vi "Main_FFT.vi"() -> ()   [LabVIEW 2026]
doc: "This template is for the Queued Message Handler design pattern.\n\nThe Event Handling Loop generates messages based on user interface actions.\n\nThe Message Handling Loop processes messages generated by the Event Handling Loop, or by other messages. The messages are string values, so new messages can be added easily to the Message Cases case structure in the Message Handling Loop. Each message cluster can also provide an optional value for Message Data, which is a variant that can be converted to whatever message-specific data is required."
uses:
  SubVIs/Controls/PCO_Config.ctl
  SubVIs/Controls/UI Data.ctl
  SubVIs/pco.labview/camera/Camera.lvclass
  SubVIs/Controls/TypeDef_FGV.ctl
  SubVIs/QMH/Message Queue/Enqueue Message (Single).vi
  SubVIs/QMH/Message Queue/Message Queue.lvlib
  SubVIs/QMH/User Event - Stop/User Event - Stop.lvlib
  SubVIs/pco.labview/pco.sdk/TimingControl/TimingControl.lvlib
panel:
  out "FFT":T1(plugin-control)
  out "Camera":T1(plugin-control)
  in  "# of frames":u16=100
  in  "SavePath":path=path "E:/exp_data/Seb"
  in  "Binning for FFT":u16(ring)=8 items=["1x1"=1, "2x2"=2, "4x4"=4, "8x8"=8]
  in  "Stop live":bool
  in  "FFT?":bool=TRUE
  in  "Grab":bool
  in  "Live":bool
  in  "PCO_Config":T2={"Exposure time (s)"=0.01, "TriggerMode"=0, "ROI X0"=1, "ROI Y0"=1, "ROI X1"=2048, "ROI Y1"=2048, "Binning"=1} {"TriggerMode" items=["auto sequence", "software trigger", "external exposure start", "external exposure control"]}
  out "Current task":string="\"Exit\" button pressed"
  in  "Exit":bool
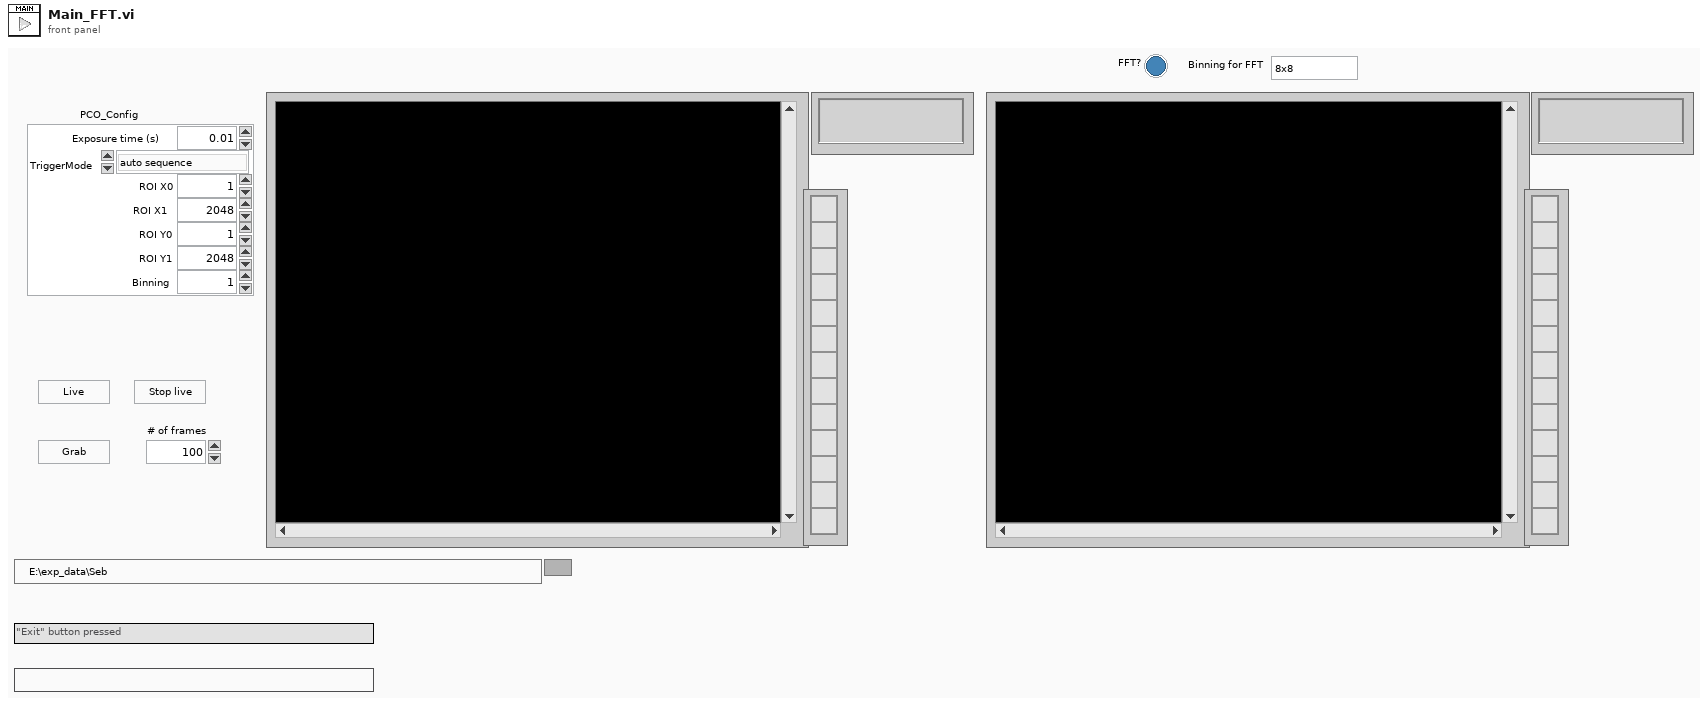
[diagram p1: front panel]
types:
  T1 = typedef "IMAQ Image.ctl" = refnum<image>
  T2 = typedef "PCO_Config.ctl" = cluster{"Exposure time (s)":dbl, "TriggerMode":u16, "ROI X0":u16, "ROI Y0":u16, "ROI X1":u16, "ROI Y1":u16, "Binning":u8}
  T3 = typedef "UI Data.ctl" = cluster{"Data Display Ref":refnum<vi>, "Exit Button Ref":refnum<vi>, "Message":string}
  T4 = typedef "Message Queue.lvlib/All Message Queues.ctl" = cluster{"UI":refnum<queue>, "Camera loop":refnum<queue>, "Display loop":refnum<queue>}
  T5 = typedef "TypeDef_FGV.ctl" = enum16{"Initialize", "Write", "Read"}
  T6 = typedef "Image Type" = u32
  T7 = enum16{"auto sequence", "software trigger", "external exposure start", "external exposure control"}
  T8 = typedef "Camera.lvclass/binning.ctl" = cluster{"vert":u16, "horz":u16, "mode":u16}
  T9 = cluster{"exposure_time_s":dbl, "delay_time_s":dbl, "roi":cluster{"x0":u64, "y0":u64, "x1":u64, "y1":u64}, "timestamp_mode":u16, "pixelrate":u32, "conversion_factor":sgl, "trigger_mode":u16, "acquire_mode":u16, "acquire_sequence_number":u32, "metadata_mode":u16, "noisefilter_mode":u16, "pixel_format":u32, "binning":T8, "auto_exposure":cluster{"region":u16, "min_exposure_s":dbl, "max_exposure_s":dbl}}
  T10 = cluster{"wSignalNum":u16, "wEnabled":u16, "wType":u16, "wPolarity":u16, "wFilterSetting":u16, "wSelected":u16, "dwParameter":u32[], "dwSignalFunctionality":u32[]}
  T11 = cluster{"wVersion":u16, "dwIMAGE_COUNTER":u32, "dwIMAGE_TIME_US":u32, "lvTimestamp":timestamp, "bIMAGE_TIME_STATUS":u8, "wEXPOSURE_TIME_BASE":u16, "dwEXPOSURE_TIME":u32, "dwFRAMERATE_MILLIHZ":u32, "sSENSOR_TEMPERATURE":i16, "wIMAGE_SIZE_X":u16, "wIMAGE_SIZE_Y":u16, "bBINNING_X":u8, "bBINNING_Y":u8, "dwSENSOR_READOUT_FREQUENCY":u32, "wSENSOR_CONV_FACTOR":u16, "dwCAMERA_SERIAL_NO":u32, "wCAMERA_TYPE":u16, "bBIT_RESOLUTION":u8, "bSYNC_STATUS":u8, "wDARK_OFFSET":u16, "bTRIGGER_MODE":u8, "bDOUBLE_IMAGE_MODE":u8, "bCAMERA_SYNC_MODE":u8, "bIMAGE_TYPE":u8, "wCOLOR_PATTERN":u16, "wCAMERA_SUBTYPE":u16, "dwEVENT_NUMBER":u32, "wIMAGE_SIZE_X_Offset":u16, "wIMAGE_SIZE_Y_Offset":u16, "bREADOUT_MODE":u8}[]
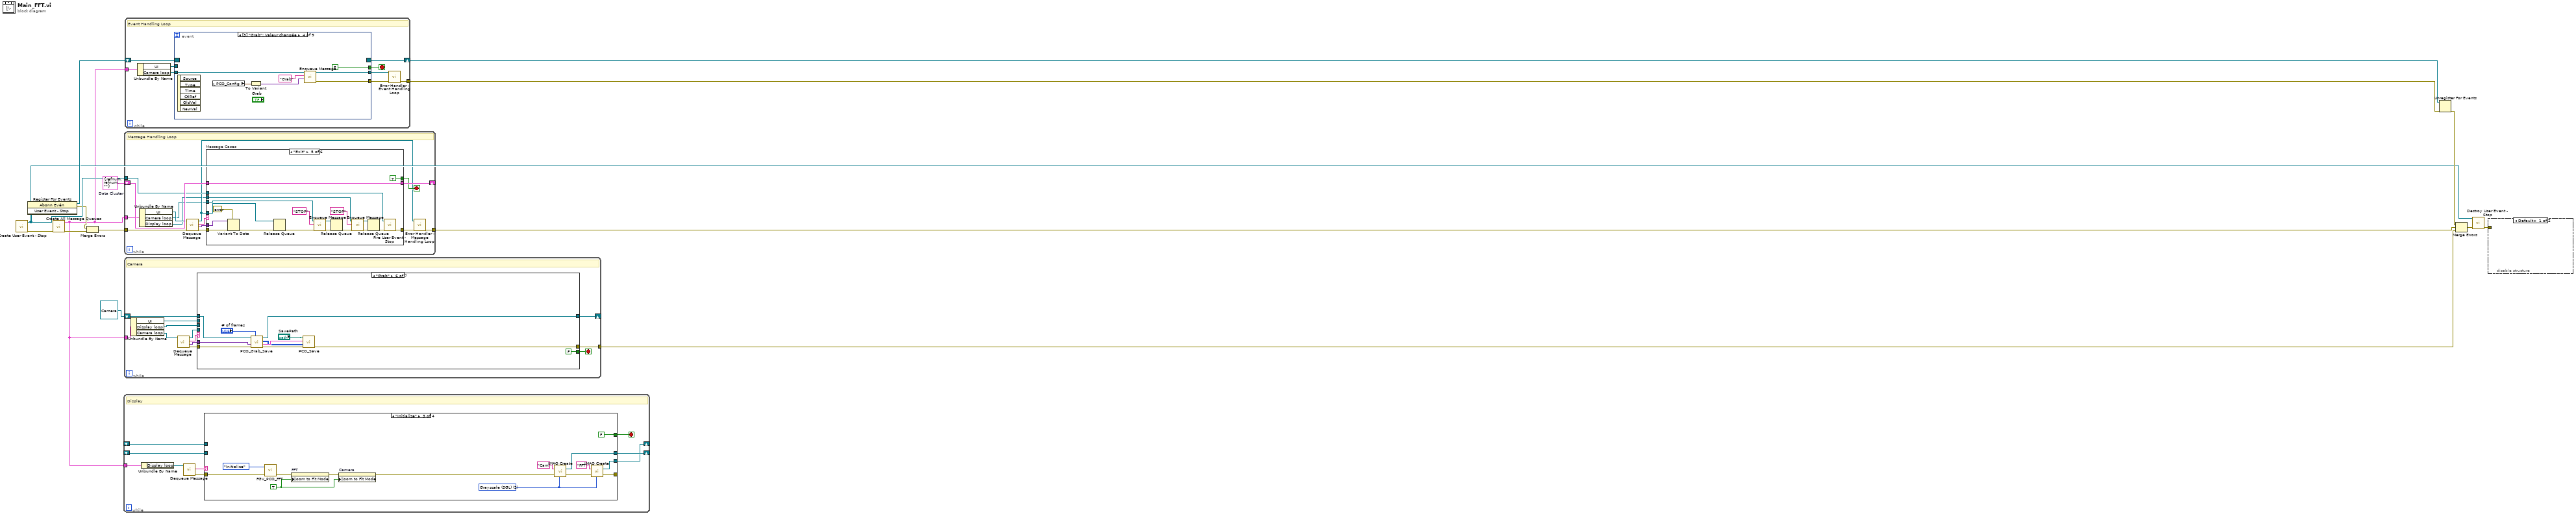
[diagram p0: block diagram]
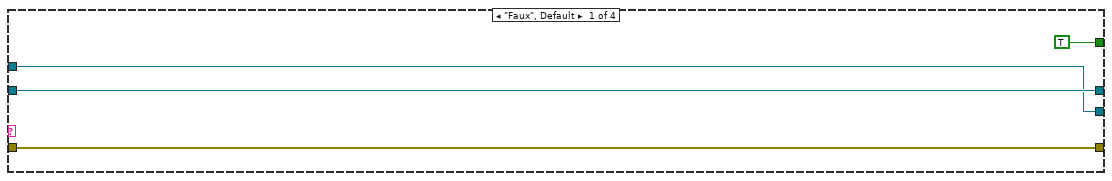
[diagram p2: hidden frame]
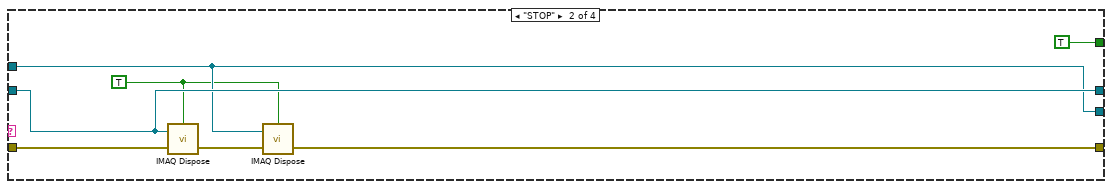
[diagram p3: hidden frame]
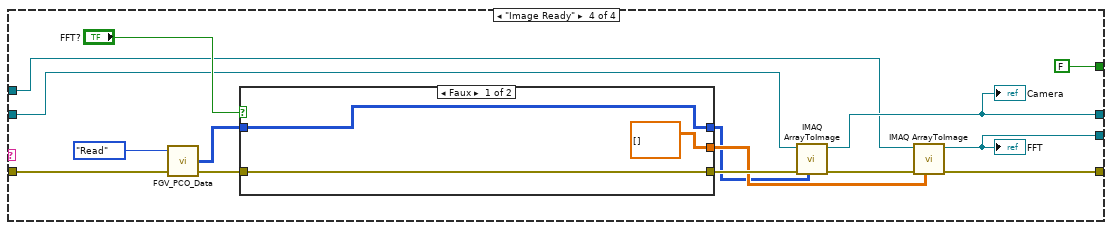
[diagram p4: hidden frame]
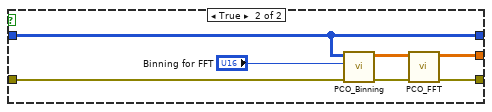
[diagram p5: hidden frame]
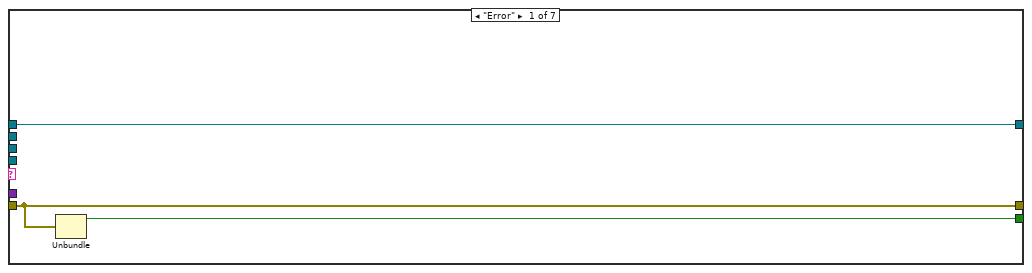
[diagram p6: hidden frame]
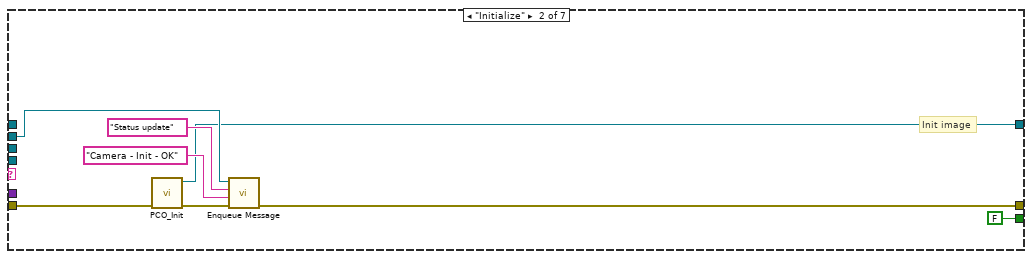
[diagram p7: hidden frame]
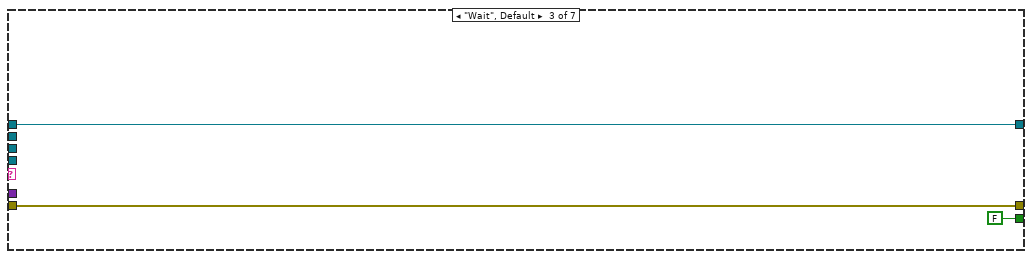
[diagram p8: hidden frame]
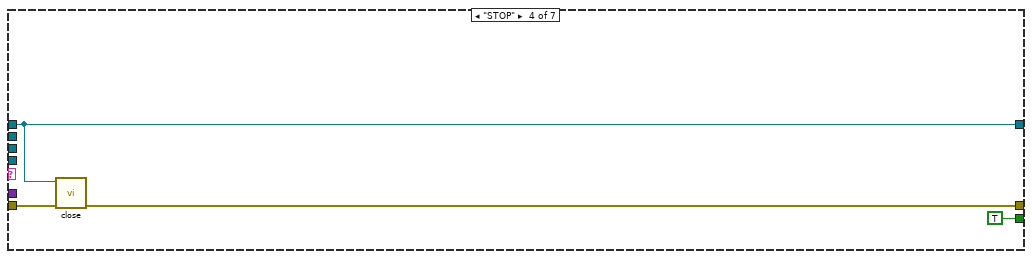
[diagram p9: hidden frame]
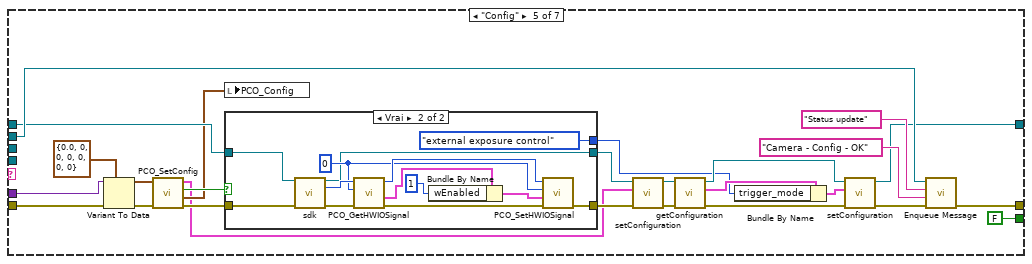
[diagram p10: hidden frame]
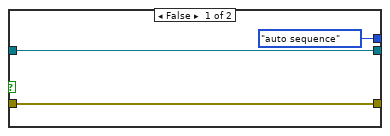
[diagram p11: hidden frame]
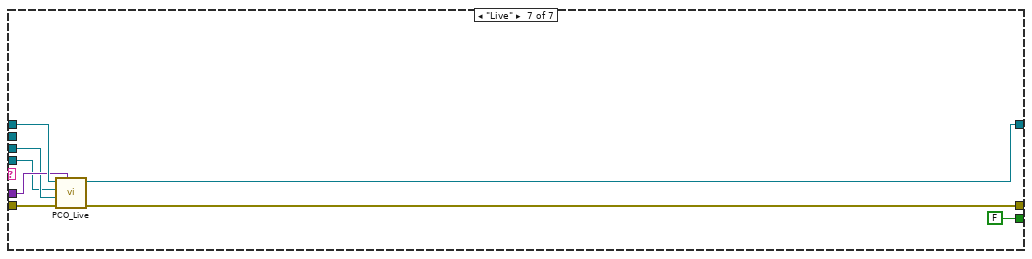
[diagram p12: hidden frame]
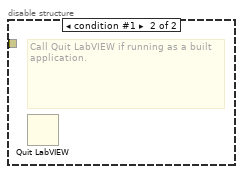
[diagram p13: hidden frame]
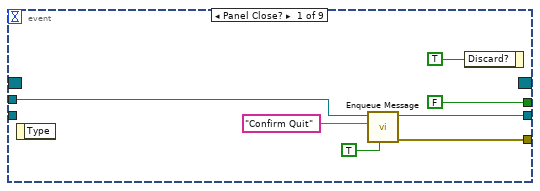
[diagram p14: hidden frame]
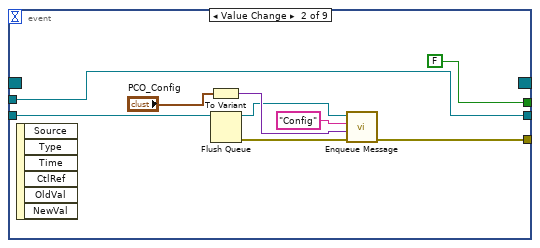
[diagram p15: hidden frame]
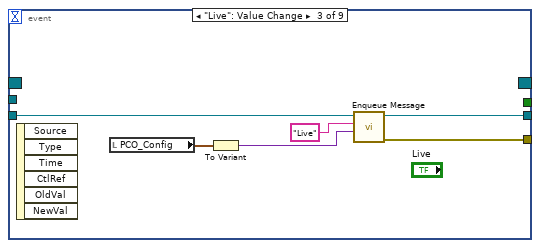
[diagram p16: hidden frame]
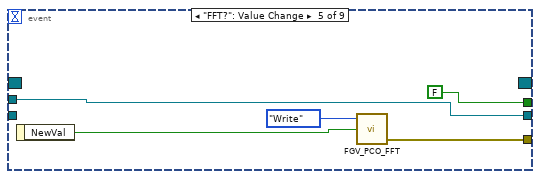
[diagram p17: hidden frame]
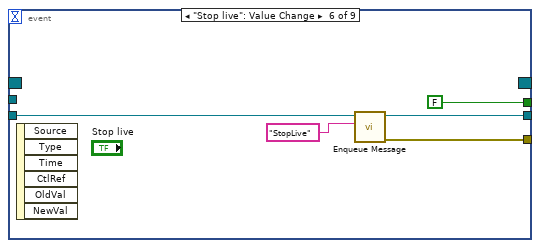
[diagram p18: hidden frame]
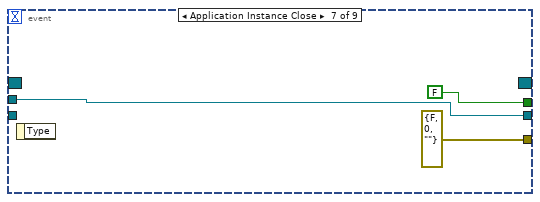
[diagram p19: hidden frame]
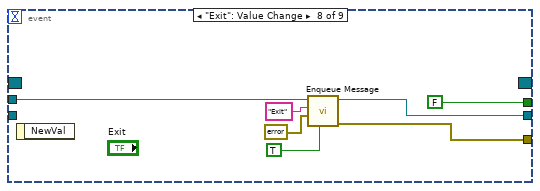
[diagram p20: hidden frame]
diagram:
  w4 = T3 {"Data Display Ref"=refnum, "Exit Button Ref"=refnum, "Message"=""}  # Data Cluster
  n1 = call "Create User Event - Stop.vi"() -> ("error out"=w14:errorcluster, "User Event - Stop"=w7:refnum<user-event>)  [unwired: 10 in]
  n2 = register-events(w7) -> (reference out=w8:refnum<event-registration>, error out=w5:errorcluster)  [unwired: 2 in]
  n3 = call "Create All Message Queues.vi"("error in (no error)"=w14) -> ("error out"=w16:errorcluster, "Message Queues out"=w2:T4)  [unwired: 9 in]
  n4 = Merge Errors(w5, w16) -> (w6:errorcluster)
  n5 = while {
    tunnel: w2 -> [w25]
    shift-right: [w20] -> _
    shift-left: _ -> [w19]
    shift-right: [w18] -> _
    shift-left: _ -> [w17]
    stop <- w21 stop-if-true
    # "Display"
    n6 = Unbundle By Name(w25) -> ("Display loop"=w24:refnum<queue>)
    n7 = call "Dequeue Message.vi"("Message Queue"=w24) -> ("error out"=w22:errorcluster, "Message"=w23:string)  [unwired: 7 in, 2 out]
    n8 = case shown="\"Initialize\"" w23 {
      tunnel: w22 -> [w29 w35 w49 w64]
      tunnel: [w29 w32 w43 w53] -> _
      tunnel: [TRUE TRUE FALSE FALSE] -> w21
      tunnel: [w27 w34 w46 w57] -> w20
      tunnel: w19 -> [w27 w34 _ w59]
      tunnel: [w26 w31 w44 w54] -> w18
      tunnel: w17 -> [w26 w31 _ w55]
      frame "Faux", Default {
      }
      frame "STOP" {
        w30 = TRUE ("All Images? (No)")
        n9 = call "IMAQ Dispose"("All Images? (No)"=w30, "Image"=w34, "error in (no error)"=w35) -> ("error out"=w33:errorcluster)  [unwired: 3 in]
        n10 = call "IMAQ Dispose"("All Images? (No)"=w30, "Image"=w31, "error in (no error)"=w33) -> ("error out"=w32:errorcluster)  [unwired: 3 in]
      }
      frame "Initialize" {
        w37 = TRUE ("Zoom to Fit Mode")
        w41 = T6 2 items=["Grayscale (U8)", "Grayscale (I16)", "Grayscale (SGL)", "Complex (CSG)", "RGB (U32)", "HSL (U32)", "RGB (U64)", "Grayscale (U16)"] ("Image Type")
        n11 = call "FGV_PCO_FFT.vi"("error in"=w49, "Action"=TypeDef_FGV."Initialize") -> ("error out"=w40:errorcluster)  [unwired: 2 in, 1 out]
        n12 = property on="FFT" class="ImageControl"(error in=w40, "Zoom to Fit Mode"=w37) -> (error out=w39:errorcluster)  [unwired: 1 in, 1 out]
        n13 = property on="Camera" class="ImageControl"(error in=w39, "Zoom to Fit Mode"=w37) -> (error out=w38:errorcluster)  [unwired: 1 in, 1 out]
        n14 = call "IMAQ Create"("Image Name"="Cam", "Image Type"=w41, "error in (no error)"=w38) -> ("New Image"=w46:T1, "error out"=w42:errorcluster)  [unwired: 2 in]
        n15 = call "IMAQ Create"("Image Name"="FFT", "Image Type"=w41, "error in (no error)"=w42) -> ("New Image"=w44:T1, "error out"=w43:errorcluster)  [unwired: 2 in]
      }
      frame "Image Ready" {
        n16 = call "FGV_PCO_Data.vi"("error in"=w64, "Action"=TypeDef_FGV."Read") -> ("error out"=w62:errorcluster, "Data"=w61:u16[][])  [unwired: 2 in]
        n17 = case shown="Faux" "FFT?" {
          tunnel: [w68 w70] -> w58
          tunnel: w62 -> [w68 w75]
          tunnel: w61 -> [w67 w72]
          tunnel: [w67 w72] -> w51
          tunnel: [dbl[][] [] ("FFT") w69] -> w52
          frame False {
          }
          frame True {
            n18 = call "PCO_Binning.vi"("error in"=w75, "Binning"="Binning for FFT", "Data"=w72) -> ("error out"=w74:errorcluster, "Data bin"=w73:dbl[][])  [unwired: 7 in]
            n19 = call "PCO_FFT.vi"("error in (no error)"=w74, "Data"=w73) -> ("error out"=w70:errorcluster, "FFT"=w69:dbl[][])  [unwired: 8 in]
          }
        }
        n20 = call "IMAQ ArrayToImage"("Image Pixels (Float)"=w51, "error in (no error)"=w58, "Image"=w59) -> ("error out"=w56:errorcluster, "Image Out"=w57:T1)  [unwired: 7 in]
        "Camera" <- w57
        n21 = call "IMAQ ArrayToImage"("Image Pixels (Float)"=w52, "error in (no error)"=w56, "Image"=w55) -> ("error out"=w53:errorcluster, "Image Out"=w54:T1)  [unwired: 7 in]
        "FFT" <- w54
      }
    }
  }
  n22 = while {
    tunnel: [w83] -> w3
    tunnel: w2 -> [w82]
    shift-right: [w80] -> _
    shift-left: refnum<class "Camera.lvclass"> refnum ("Camera out") -> [w79]
    stop <- w84 stop-if-true
    # "Camera"
    n23 = Unbundle By Name(w82) -> ("UI"=w81:refnum<queue>, "Display loop"=w77:refnum<queue>, "Camera loop"=w76:refnum<queue>)
    n24 = call "Dequeue Message.vi"("Message Queue"=w76) -> ("error out"=w87:errorcluster, "Message Data"=w85:variant, "Message"=w86:string, "dup Message Queue"=w78:refnum<queue>)  [unwired: 7 in]
    n25 = case shown="\"Grab\"" w86 {
      tunnel: w87 -> [w90 w94 w101 w104 w130 w155 w164]
      tunnel: w85 -> [_ _ _ _ w129 w154 w163]
      tunnel: w81 -> [_ w98 _ _ w125 _ _]
      tunnel: [w89 FALSE ("status") FALSE ("status") TRUE FALSE ("status") FALSE ("status") FALSE ("status")] -> w84
      tunnel: [w90 w92 w101 w103 w124 w148 w161] -> w83
      tunnel: w78 -> [_ _ _ _ _ _ w159]
      tunnel: [w88 w93 w100 w102 w112 w158 w160] -> w80
      tunnel: w79 -> [w88 _ w100 w102 w120 w153 w165]
      tunnel: w77 -> [_ _ _ _ _ _ w162]
      frame "Error" {
        n26 = Unbundle(w90) -> ("status"=w89:bool)  [unwired: 2 out]
      }
      frame "Initialize" {
        # "Init image"
        n27 = call "PCO_Init.vi"("entrée d'erreur (pas d'erreur)"=w94) -> ("sortie d'erreur"=w91:errorcluster, "Camera en sortie"=w93:refnum<class "Camera.lvclass">)  [unwired: 9 in]
        n28 = call-poly "Enqueue Message.vi"("error in (no error)"=w91, "Message Data"="Camera - Init - OK", "Message"="Status update", "Message Queue"=w98) -> ("error out"=w92:errorcluster)  [unwired: 6 in, 1 out]
      }
      frame "Wait", Default {
      }
      frame "STOP" {
        n29 = call-dynamic "close.vi"("error in (no error)"=w104, "Camera in"=w102) -> ("error out"=w103:errorcluster)  [unwired: 9 in]
      }
      frame "Config" {
        n30 = Variant To Data(error in=w130, type=T2 {"Exposure time (s)"=0.0, "TriggerMode"=0, "ROI X0"=0, "ROI Y0"=0, "ROI X1"=0, "ROI Y1"=0, "Binning"=0} ("PCO_Config"), Variant=w129) -> (data=w127:T2, error out=w117:errorcluster)
        n31 = call "PCO_SetConfig.vi"("error in"=w117, "PCO_Config"=w127) -> ("error out"=w116:errorcluster, "PCO_Config 2"=w114:T2, "Trigger externe?"=w118:bool, "configuration"=w106:T9)  [unwired: 6 in]
        n32 = local write "PCO_Config"(w114) -> ()
        n33 = case shown="Vrai" w118 {
          tunnel: w116 -> [w134 w140]
          tunnel: [w134 w135] -> w121
          tunnel: w120 -> [w133 w138]
          tunnel: [w133 w137] -> w119
          tunnel: [T7."auto sequence" ("TriggerMode") T7."external exposure control" ("TriggerMode")] -> w107
          frame False {
          }
          frame True {
            w142 = u16 0 ("wSignalNum")
            n34 = call-dynamic "sdk.vi"("Camera in"=w138, "error in (no error)"=w140) -> ("Camera out"=w137:refnum<class "Camera.lvclass">, "sdk"=w143:u64, "error out"=w139:errorcluster)  [unwired: 11 in]
            n35 = call "PCO_GetHWIOSignal.vi"("error in (no error)"=w139, "wSignalNum"=w142, "ph"=w143) -> ("error out"=w145:errorcluster, "strSignal"=w147:T10, "ph out"=w144:u64)  [unwired: 5 in, 1 out]
            n36 = Bundle By Name(cluster=w147, "wEnabled"=u16 1) -> (w146:T10)
            n37 = call "PCO_SetHWIOSignal.vi"("error in (no error)"=w145, "strSignal"=w146, "wSignalNum"=w142, "ph"=w144) -> ("error out"=w135:errorcluster)  [unwired: 5 in, 2 out]
          }
        }
        n38 = call-dynamic "setConfiguration.vi"("error in (no error)"=w121, "configuration"=w106, "Camera in"=w119) -> ("error out"=w115:errorcluster, "Camera out"=w122:refnum<class "Camera.lvclass">)  [unwired: 7 in]
        n39 = call-dynamic "getConfiguration.vi"("error in (no error)"=w115, "Camera in"=w122) -> ("error out"=w111:errorcluster, "configuration"=w109:T9, "Camera out"=w113:refnum<class "Camera.lvclass">)  [unwired: 7 in]
        n40 = Bundle By Name(cluster=w109, "trigger_mode"=w107) -> (w108:T9)
        n41 = call-dynamic "setConfiguration.vi"("error in (no error)"=w111, "configuration"=w108, "Camera in"=w113) -> ("error out"=w110:errorcluster, "Camera out"=w112:refnum<class "Camera.lvclass">)  [unwired: 7 in]
        n42 = call-poly "Enqueue Message.vi"("error in (no error)"=w110, "Message Data"="Camera - Config - OK", "Message"="Status update", "Message Queue"=w125) -> ("error out"=w124:errorcluster)  [unwired: 6 in, 1 out]
      }
      frame "Grab" {
        n43 = call "PCO_Grab_Save.vi"("# of frames"="# of frames", "entrée d'erreur (pas d'erreur)"=w155, "Message Data"=w154, "Camera en entrée"=w153) -> ("sortie d'erreur"=w151:errorcluster, "meta_data_list"=w150:T11, "Raw data (U16)"=w149:u16[][][], "Camera en sortie"=w158:refnum<class "Camera.lvclass">)  [unwired: 4 in]
        n44 = call "PCO_Save.vi"("entrée d'erreur (pas d'erreur)"=w151, "raw_image_list (U16)"=w149, "meta_data_list"=w150, "SavePath"="SavePath") -> ("sortie d'erreur"=w148:errorcluster)  [unwired: 7 in]
      }
      frame "Live" {
        n45 = call "PCO_Live.vi"("Message Data"=w163, "entrée d'erreur (pas d'erreur)"=w164, "Display loop"=w162, "dup Message Queue"=w159, "Camera en entrée"=w165) -> ("sortie d'erreur"=w161:errorcluster, "Camera en sortie"=w160:refnum<class "Camera.lvclass">)  [unwired: 5 in]
      }
    }
  }
  n46 = while {
    shift-right: [w180] -> _
    shift-left: w4 -> [w181]
    tunnel: w7 -> [w178]
    tunnel: w6 -> [w177]
    tunnel: [w172] -> w15
    tunnel: w2 -> [w170]
    stop <- w179 stop-if-true
    # "Message Handling Loop"
    n47 = Unbundle By Name(w170) -> ("UI"=w169:refnum<queue>, "Camera loop"=w168:refnum<queue>, "Display loop"=w167:refnum<queue>)
    n48 = call "Dequeue Message.vi"("error in (no error)"=w177, "Message Queue"=w169) -> ("error out"=w176:errorcluster, "Message Data"=w174:variant, "Message"=w175:string, "dup Message Queue"=w173:refnum<queue>)  [unwired: 6 in]
    n49 = case "Message Cases" shown="\"Exit\"" w175 {
      tunnel: w173 -> [w184 _ _ w206 w220 _]
      tunnel: w176 -> [w189 w195 w202 w208 w221 w229]
      tunnel: [w190 w192 w197 w203 w216 w229] -> w171
      tunnel: w181 -> [w188 w196 w201 w207 w228 w230]
      tunnel: [w187 w196 w201 w207 w228 w230] -> w180
      tunnel: [_ _ _ _ TRUE _] -> w179
      tunnel: w174 -> [_ w194 w200 _ w224 _]
      tunnel: w178 -> [_ _ _ _ w226 _]
      tunnel: w168 -> [_ _ _ _ w219 _]
      tunnel: w167 -> [_ _ _ _ w209 _]
      frame "Initialize" {
        w182 = "Initial Message" ("Initial Message")
        n50 = control-ref of="Current task"() -> (w183:refnum<vi>)
        n51 = control-ref of="Exit"() -> (w186:refnum<vi>)
        n52 = Bundle By Name(cluster=w188, "Data Display Ref"=w183, "Exit Button Ref"=w186, "Message"=w182) -> (w187:T3)
        n53 = call-poly "Enqueue Message.vi"("error in (no error)"=w189, "Message Data"=w182, "Message"="Update Display", "Message Queue"=w184) -> ("error out"=w190:errorcluster)  [unwired: 6 in, 1 out]
      }
      frame "Update Display" {
        n54 = Variant To Data(error in=w195, type="", Variant=w194) -> (data=→"Current task":string, error out=w192:errorcluster)
      }
      frame "Error" {
        n55 = Variant To Data(error in=w202, type=errorcluster {"status"=FALSE, "code"=0, "source"=""} ("error constant"), Variant=w200) -> (data=w198:errorcluster, error out=w197:errorcluster)
        n56 = call <vilib>:"Simple Error Handler.vi"("error in (no error)"=w198) -> ()  [unwired: 4 in, 5 out]
      }
      frame "Confirm Quit" {
        n57 = call-poly "Enqueue Message.vi"("Priority Message? (F)"=TRUE, "error in (no error)"=w208, "Message"="Exit", "Message Queue"=w206) -> ("error out"=w203:errorcluster)  [unwired: 6 in, 1 out]
      }
      frame "Exit" {
        n58 = Variant To Data(error in=w221, type=errorcluster {"status"=FALSE, "code"=0, "source"=""} ("error constant"), Variant=w224) -> (error out=w217:errorcluster)  [unwired: 1 out]
        n59 = Release Queue(queue=w220, error in (no error)=w217) -> (error out=w215:errorcluster)  [unwired: 1 in, 2 out]
        n60 = call-poly "Enqueue Message.vi"("error in (no error)"=w215, "Message"="STOP", "Message Queue"=w219) -> ("error out"=w223:errorcluster, "dup Message Queue"=w222:refnum<queue>)  [unwired: 7 in]
        n61 = Release Queue(queue=w222, error in (no error)=w223) -> (error out=w211:errorcluster)  [unwired: 1 in, 2 out]
        n62 = call-poly "Enqueue Message.vi"("error in (no error)"=w211, "Message"="STOP", "Message Queue"=w209) -> ("error out"=w212:errorcluster, "dup Message Queue"=w213:refnum<queue>)  [unwired: 7 in]
        n63 = Release Queue(queue=w213, error in (no error)=w212) -> (error out=w210:errorcluster)  [unwired: 1 in, 2 out]
        n64 = call "Fire User Event - Stop.vi"("error in (no error)"=w210, "User Event - Stop"=w226) -> ("error out"=w216:errorcluster)  [unwired: 9 in]
      }
      frame Default {
      }
    }
    n65 = call "Error Handler - Message Handling Loop.vi"("error in (no error)"=w171, "Message Queue"=w173) -> ("dup error in"=w172:errorcluster)  [unwired: 8 in, 1 out]
  }
  n66 = while {
    shift-right: [w238] -> w11
    shift-left: w8 -> [w239]
    tunnel: [w234] -> w9
    tunnel: w2 -> [w231]
    stop <- w236 stop-if-true
    # "Event Handling Loop"
    n67 = Unbundle By Name(w231) -> ("UI"=w233:refnum<queue>, "Camera loop"=w232:refnum<queue>)
    n68 = event shown="[3] \"Grab\": Valeur changée" {
      selector: w239 -> [_ _ _ _ _ _ _ _ _]
      dyn-events: [_ _ _ _ _ _ _ _ _] -> w238
      timeout: _ -> [_ _ _ _ _ _ _ _ _]
      tunnel: [FALSE ("Discard?") FALSE ("Discard?") _ FALSE ("Discard?") FALSE ("Discard?") FALSE ("Discard?") FALSE ("Discard?") FALSE ("Discard?") TRUE ("Discard?")] -> w236
      tunnel: w233 -> [w245 w255 _ _ w273 _ w281 w288 w292]
      tunnel: [w244 w251 w258 w265 w271 w276 errorcluster {"status"=FALSE, "code"=0, "source"=""} ("error out") w282 errorcluster {"status"=FALSE, "code"=0, "source"=""} ("error out")] -> w237
      tunnel: [w243 w255 w257 w266 w273 w275 w281 w287 w292] -> w235
      tunnel: w232 -> [_ w249 w256 w267 _ w277 _ _ _]
      event Panel Close? {
        n69 = event-data() -> ()  [unwired: 1 in, 1 out]
        n70 = call-poly "Enqueue Message.vi"("Priority Message? (F)"=TRUE, "Message"="Confirm Quit", "Message Queue"=w245) -> ("error out"=w244:errorcluster, "dup Message Queue"=w243:refnum<queue>)  [unwired: 7 in]
        n71 = event-data("Discard?"=TRUE) -> ()  [unwired: 1 in, 1 out]
      }
      event Value Change {
        n72 = event-data() -> ()  [unwired: 1 in, 6 out]
        n73 = To Variant(anything="PCO_Config") -> (Variant=w252:variant)
        n74 = Flush Queue(queue=w249) -> (queue out=w247:refnum<queue>, error out=w248:errorcluster)  [unwired: 1 in, 1 out]
        n75 = call-poly "Enqueue Message.vi"("error in (no error)"=w248, "Message Data"=w252, "Message"="Config", "Message Queue"=w247) -> ("error out"=w251:errorcluster)  [unwired: 6 in, 1 out]
      }
      event "Live": Value Change {
        n76 = event-data() -> ()  [unwired: 1 in, 6 out]
        n77 = local read "PCO_Config"() -> (w261:T2)
        n78 = To Variant(anything=w261) -> (Variant=w260:variant)
        n79 = call-poly "Enqueue Message.vi"("Message Data"=w260, "Message"="Live", "Message Queue"=w256) -> ("error out"=w258:errorcluster, "dup Message Queue"=w257:refnum<queue>)  [unwired: 7 in]
      }
      event "Grab": Value Change {
        n80 = event-data() -> ()  [unwired: 1 in, 6 out]
        n81 = local read "PCO_Config"() -> (w263:T2)
        n82 = To Variant(anything=w263) -> (Variant=w262:variant)
        n83 = call-poly "Enqueue Message.vi"("Message Data"=w262, "Message"="Grab", "Message Queue"=w267) -> ("error out"=w265:errorcluster, "dup Message Queue"=w266:refnum<queue>)  [unwired: 7 in]
      }
      event "FFT?": Value Change {
        n84 = event-data() -> ("NewVal"=w269:bool)  [unwired: 1 in]
        n85 = call "FGV_PCO_FFT.vi"("FFT?"=w269, "Action"=TypeDef_FGV."Write") -> ("error out"=w271:errorcluster)  [unwired: 2 in, 1 out]
      }
      event "Stop live": Value Change {
        n86 = event-data() -> ()  [unwired: 1 in, 6 out]
        n87 = call-poly "Enqueue Message.vi"("Message"="StopLive", "Message Queue"=w277) -> ("error out"=w276:errorcluster, "dup Message Queue"=w275:refnum<queue>)  [unwired: 8 in]
      }
      event Application Instance Close {
        n88 = event-data() -> ()  [unwired: 1 in, 1 out]
      }
      event "Exit": Value Change {
        n89 = event-data() -> ()  [unwired: 1 in, 1 out]
        n90 = call-poly "Enqueue Message.vi"("Priority Message? (F)"=TRUE, "Message Data"=errorcluster {"status"=FALSE, "code"=0, "source"=""} ("error constant"), "Message"="Exit", "Message Queue"=w288) -> ("error out"=w282:errorcluster, "dup Message Queue"=w287:refnum<queue>)  [unwired: 6 in]
      }
      event User Event {
        n91 = event-data() -> ()  [unwired: 1 in, 1 out]
        n92 = local write "Current task"("\"Exit\" button pressed" ("VI Stopped")) -> ()
      }
    }
    n93 = call "Error Handler - Event Handling Loop.vi"("error in (no error)"=w237, "Message Queue"=w235) -> ("dup error in"=w234:errorcluster)  [unwired: 8 in, 1 out]
  }
  n94 = Unregister For Events(event registration refnum=w11, error in=w9) -> (error out=w12:errorcluster)
  n95 = Merge Errors(w12, w15, w3) -> (w13:errorcluster)
  n96 = call "Destroy User Event - Stop.vi"("error in (no error)"=w13, "User Event - Stop"=w7) -> ("error out"=w10:errorcluster)  [unwired: 9 in]
  n97 = disable-structure shown="Default" {
    disable-tunnel: w10 -> [_ _]
    frame condition #0 (active) {
    }
    frame condition #1 {
      # "Call Quit LabVIEW if running as a built application."
      n98 = Quit LabVIEW() -> ()  [unwired: 1 in]
    }
  }
